vi "startUEFGV.vi"(8 "error in (no error)":errorcluster, 11 "Enum":T1) -> (0 "error out":errorcluster, 3 "Start User Event":refnum<user-event>)   [LabVIEW 2017, in "programControl.lvlib"]
uses:
  programControl.lvlib
  TypeDefs/UEFGVcontrol.ctl
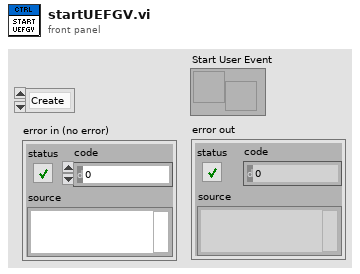
[diagram p1: front panel]
types:
  T1 = typedef "UEFGVcontrol.ctl" = enum16{"Create", "Get", "Destroy"}
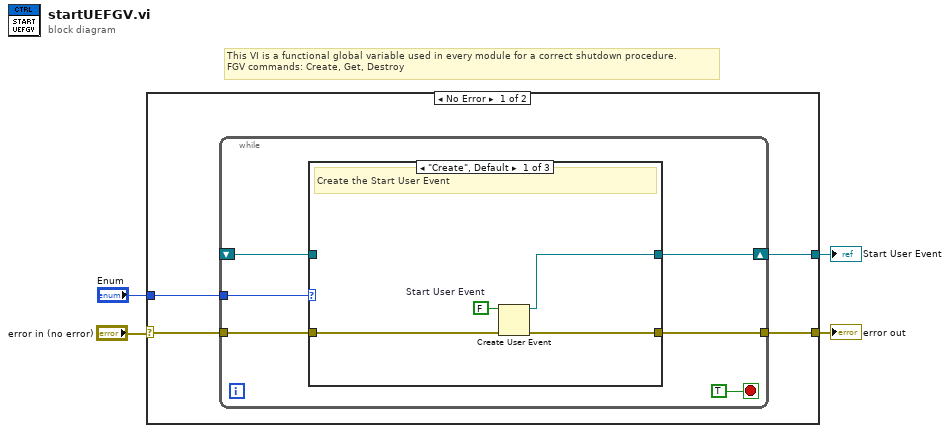
[diagram p0: block diagram]
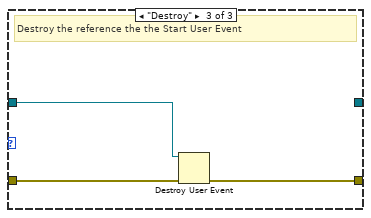
[diagram p3: hidden frame]
diagram:
  # "This VI is a functional global variable used in every module for a correct shutdown procedure.\nFGV commands: Create, Get, Destroy"
  n1 = case shown="No Error" "error in (no error)" {
    selector: "error in (no error)" -> [w7 w24]
    tunnel: [w6 w24] -> w3
    tunnel: "Enum" -> [w8 _]
    tunnel: [w5 _] -> w2
    frame No Error {
      n2 = while {
        tunnel: w8 -> [w14]
        tunnel: w7 -> [w13]
        tunnel: [w11] -> w6
        shift-right: [w10] -> w5
        shift-left: _ -> [w9]
        stop <- TRUE stop-if-true
        n3 = case shown="\"Create\", Default" w14 {
          tunnel: w13 -> [w18 w20 w23]
          tunnel: [w17 w20 w22] -> w11
          tunnel: [w16 w19 _] -> w10
          tunnel: w9 -> [_ w19 w21]
          frame "Create", Default {
            w15 = FALSE  # Start User Event
            # "Create the Start User Event"
            n4 = Create User Event(user event datatype=w15, error in=w18) -> (user event=w16:refnum<user-event>, error out=w17:errorcluster)
          }
          frame "Get" {
            # "Obtain a reference the the UE"
          }
          frame "Destroy" {
            # "Destroy the reference the the Start User Event"
            n5 = Destroy User Event(user event=w21, error in=w23) -> (error out=w22:errorcluster)
          }
        }
      }
    }
    frame Error {
    }
  }
  "error out" <- w3
  "Start User Event" <- w2
